vi "get_consecutive_repetitions.vi"(8 "error in (no error)":errorcluster, 11 "ImagingModeDL090130Frame in":refnum<class "ImagingModeDL090130Frame.lvclass">=refnum) -> (0 "error out":errorcluster, 2 "number of consecutive repetitions":i32, 3 "ImagingModeDL090130Frame out":refnum<class "ImagingModeDL090130Frame.lvclass">)   [LabVIEW 2010, in "ImagingModeDL090130Frame.lvclass"]
uses:
  ImagingModeDL090130Frame.lvclass
  ImagingModeDL090130Frame.lvclass/ImagingModeDL090130Frame.ctl
panel:
  # "Note that this method returns the number of consecutive repetitions for single-sweep/experiment mode.\n\nI.e., it does NOT return -1 for free-run mode (reason: if we switch between run modes, the other top-level components are not instructed anymore by the ImagingMode, rather they have to figure out the actual value by themselves."
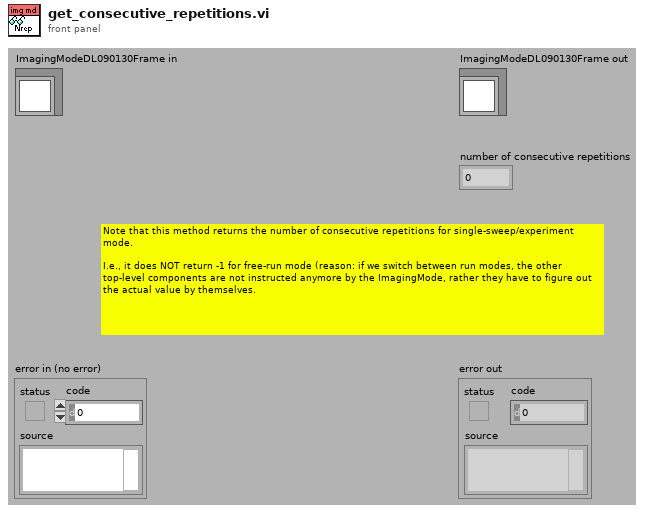
[diagram p1: front panel]
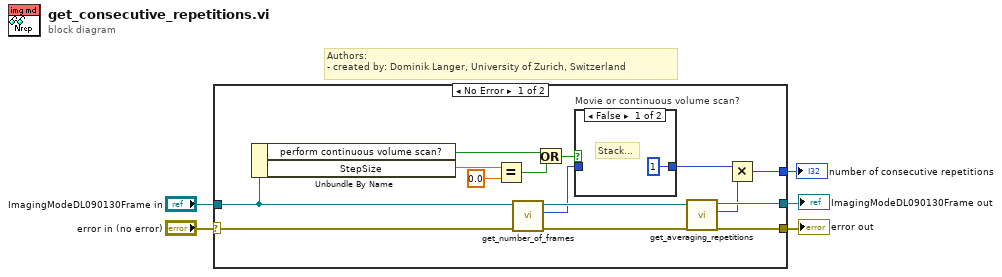
[diagram p0: block diagram]
diagram:
  # "Authors: \n- created by: Dominik Langer, University of Zurich, Switzerland"
  n1 = case shown="No Error" "error in (no error)" {
    selector: "error in (no error)" -> [w16 w24]
    tunnel: [w20 w24] -> w4
    tunnel: [w19 w23] -> w2
    tunnel: "ImagingModeDL090130Frame in" -> [w15 w23]
    tunnel: [w18 _] -> w1
    frame No Error {
      n2 = Unbundle By Name(w15) -> ("perform continuous volume scan?"=w7:bool, "StepSize"=w17:dbl[unit])
      n3 = Equal?(x=w17, y=dbl[unit] 0.0) -> (x = y?=w9:bool)
      n4 = call-dynamic "get_number_of_frames.vi"("error in (no error)"=w16, "ImagingModeDL090130Frame in"=w15) -> ("error out"=w13:errorcluster, "number of frames"=w6:i32, "ImagingModeDL090130Frame out"=w14:refnum<class "ImagingModeDL090130Frame.lvclass">)  [unwired: 7 out]
      n5 = Or(x=w7, y=w9) -> (x .or. y?=w8:bool)
      n6 = case "Movie or continuous volume scan?" shown="False" w8 {
        tunnel: [1 ("number of frames") w22] -> w12
        tunnel: w6 -> [_ w22]
        frame False {
          # "Stack..."
        }
        frame True {
          # "Movie..."
        }
      }
      n7 = call-dynamic "get_averaging_repetitions.vi"("error in (no error)"=w13, "ImagingModeDL090130Frame in"=w14) -> ("error out"=w20:errorcluster, "averaging repetitions"=w11:i32, "ImagingModeDL090130Frame out"=w19:refnum<class "ImagingModeDL090130Frame.lvclass">)  [unwired: 7 out]
      n8 = Multiply(x=w12, y=w11) -> (x*y=w18:i32)
    }
    frame Error {
    }
  }
  "error out" <- w4
  "ImagingModeDL090130Frame out" <- w2
  "number of consecutive repetitions" <- w1
